vi "LSCI332ReadCalib.vi"(0 "VISA Rsrc":refnum<visa-resource-name>="GPIB0::12::INSTR" caption="Adresse du contrôlleur", 2 "No Courbe":u32=21 min=1 max=41 step=1, 11 "error in":errorcluster) -> (3 "Nom":string="CourbeTest", 4 "ValCalib":dbl[][](array[numeric]) caption="Valeurs de Calibration", 6 "No de série":string="Standard", 8 "Coefficient":u16(ring)=2 items=["Faites un choix", "négatif", "positif"], 10 "Format":u16(ring)=2 items=["Faites un choix", "mV/K", "V/K", "Ohm/K", "log Ohm/K"], 14 "TLim":dbl=475.0 caption="T° de Contrôle Max (K)", 15 "error out":errorcluster)   [LabVIEW 2012]
doc: "Ce Vi écrit l'entête et les points d'une courbe de calibration dans l'emplacement spécifié du contrôlleur de température"
panel:
  # "Température (K)"
  # "Sortie Capteur"
  # "+5"
  # "+10"
  # "+15"
  # "+20"
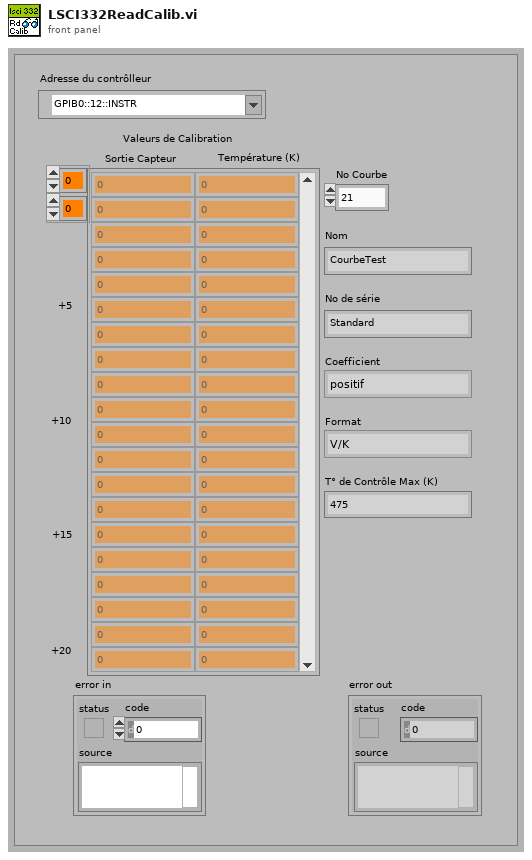
[diagram p1: front panel]
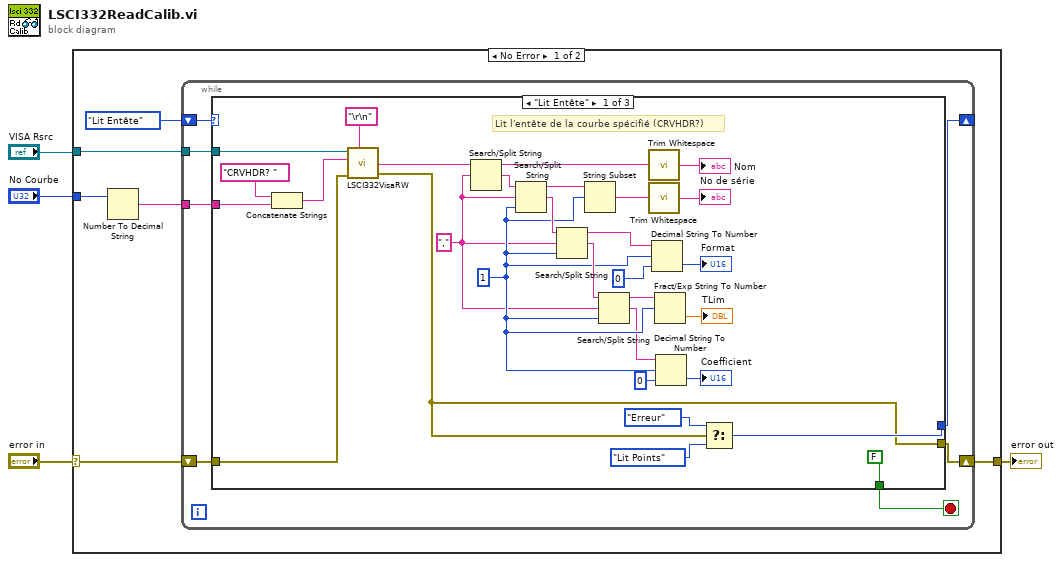
[diagram p0: block diagram]
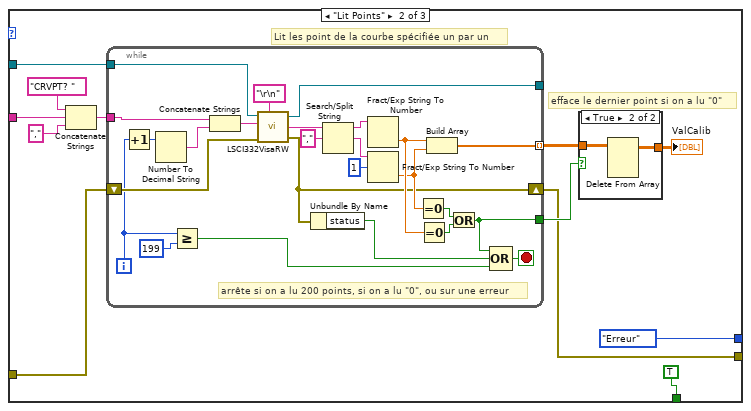
[diagram p2: hidden frame]
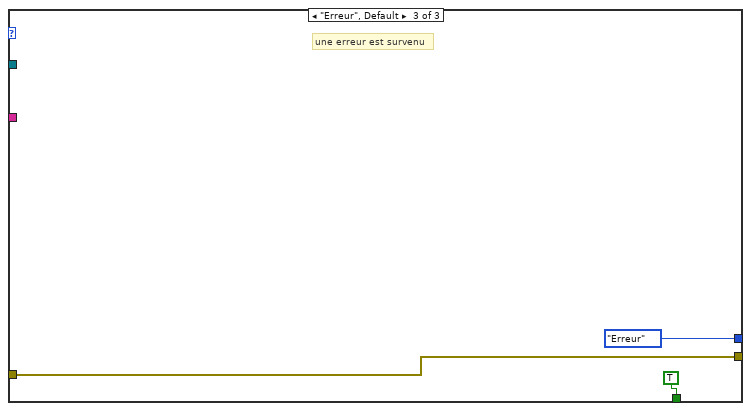
[diagram p4: hidden frame]
diagram:
  n1 = case shown="No Error" "error in" {
    selector: "error in" -> [w10 w91]
    tunnel: "VISA Rsrc" -> [w7 _]
    tunnel: "No Courbe" -> [w9 _]
    tunnel: [w6 w91] -> w1
    frame No Error {
      n2 = Number To Decimal String(number=w9) -> (decimal integer string=w8:string)  [unwired: 1 in]
      n3 = while {
        shift-right: [w11] -> w6
        shift-left: w10 -> [w17]
        tunnel: w8 -> [w15]
        tunnel: w7 -> [w14]
        shift-right: [w12] -> _
        shift-left: enum16{"Lit Entête", "Lit Points", "Erreur"}."Lit Entête" -> [w13]
        stop <- w16 stop-if-true
        n4 = case shown="\"Lit Entête\"" w13 {
          tunnel: w17 -> [w42 w54 w88]
          tunnel: [FALSE TRUE TRUE] -> w16
          tunnel: w15 -> [w45 w55 _]
          tunnel: w14 -> [w43 w56 _]
          tunnel: [w20 enum16{"Lit Entête", "Lit Points", "Erreur"}."Erreur" enum16{"Lit Entête", "Lit Points", "Erreur"}."Erreur"] -> w12
          tunnel: [w19 w50 w88] -> w11
          frame "Lit Entête" {
            w18 = ","
            w26 = 1
            # "Lit l'entête de la courbe spécifié (CRVHDR?)"
            n5 = Concatenate Strings("CRVHDR? ", w45) -> (w44:string)
            n6 = call <userlib>:"LSCI332VisaRW.vi"("error in (no error)"=w42, "EOS (Aucun)"="\r\n", "ChaineCom"=w44, "VISA Rsrc"=w43) -> ("error out"=w19:errorcluster, "ChaineRep"=w39:string)  [unwired: 3 in, 2 out]
            n7 = Search/Split String(string=w39, search string/char (-)=w18) -> (substring before match=w32:string, match + rest of string=w40:string)  [unwired: 1 in, 1 out]
            n8 = Search/Split String(string=w40, search string/char (-)=w18, offset (0)=w26) -> (substring before match=w38:string, match + rest of string=w41:string)  [unwired: 1 out]
            n9 = Search/Split String(string=w41, search string/char (-)=w18, offset (0)=w26) -> (substring before match=w37:string, match + rest of string=w34:string)  [unwired: 1 out]
            n10 = String Subset(string=w38, offset (0)=w26) -> (substring=w30:string)  [unwired: 1 in]
            n11 = Search/Split String(string=w34, search string/char (-)=w18, offset (0)=w26) -> (substring before match=w33:string, match + rest of string=w25:string)  [unwired: 1 out]
            n12 = call <vilib>:"Trim Whitespace.vi"("string"=w32) -> ("trimmed string"=→"Nom":string)  [unwired: 1 in]
            n13 = call <vilib>:"Trim Whitespace.vi"("string"=w30) -> ("trimmed string"=→"No de série":string)  [unwired: 1 in]
            n14 = Decimal String To Number(string=w37, offset=w26, default (0L)=u16 0 ("default (0 I32)")) -> (number=→"Format":u16)  [unwired: 1 out]
            n15 = Fract/Exp String To Number(string=w33, offset=w26) -> (number=→"TLim":dbl)  [unwired: 2 in, 1 out]
            n16 = Decimal String To Number(string=w25, offset=w26, default (0L)=u16 0 ("default (0 I32)")) -> (number=→"Coefficient":u16)  [unwired: 1 out]
            n17 = Select(t=enum16{"Lit Entête", "Lit Points", "Erreur"}."Erreur", s=w19, f=enum16{"Lit Entête", "Lit Points", "Erreur"}."Lit Points") -> (s? t:f=w20:enum16{"Lit Entête", "Lit Points", "Erreur"})
          }
          frame "Lit Points" {
            # "Lit les point de la courbe spécifiée un par un"
            # "efface le dernier point si on a lu \"0\""
            n18 = Concatenate Strings("CRVPT? ", w55, ",") -> (w58:string)
            n19 = while {
              tunnel: w58 -> [w87]
              tunnel: w56 -> [w85]
              shift-right: [w65] -> w50
              shift-left: w54 -> [w84]
              tunnel: [w71] -> w53 mode=indexing
              tunnel: [w77] -> _
              tunnel: [w66] -> w51
              i -> [w75]
              stop <- w72 stop-if-true
              # "arrête si on a lu 200 points, si on a lu \"0\", ou sur une erreur"
              n20 = Increment(x=w75) -> (x+1=w74:i32)
              n21 = Number To Decimal String(number=w74) -> (decimal integer string=w73:string)  [unwired: 1 in]
              n22 = Greater Or Equal?(x=w75, y=199) -> (x >= y?=w64:bool)
              n23 = Concatenate Strings(w87, w73) -> (w86:string)
              n24 = call <userlib>:"LSCI332VisaRW.vi"("error in (no error)"=w84, "EOS (Aucun)"="\r\n", "ChaineCom"=w86, "VISA Rsrc"=w85) -> ("error out"=w65:errorcluster, "ChaineRep"=w82:string, "VISA Rsrc Out"=w77:refnum<visa-resource-name>)  [unwired: 3 in, 1 out]
              n25 = Unbundle By Name(w65) -> ("status"=w63:bool)
              n26 = Search/Split String(string=w82, search string/char (-)=",") -> (substring before match=w80:string, match + rest of string=w79:string)  [unwired: 1 in, 1 out]
              n27 = Fract/Exp String To Number(string=w80) -> (number=w70:dbl)  [unwired: 3 in, 1 out]
              n28 = Fract/Exp String To Number(string=w79, offset=1) -> (number=w69:dbl)  [unwired: 2 in, 1 out]
              n29 = Equal To 0?(x=w69) -> (x = 0?=w67:bool)
              n30 = Equal To 0?(x=w70) -> (x = 0?=w68:bool)
              n31 = Build Array(w70, w69) -> (w71:dbl[])
              n32 = Or(x=w67, y=w68) -> (x .or. y?=w66:bool)
              n33 = Compound Arithmetic op=OR(w66, w63, w64) -> (w72:bool)
            }
            n34 = case shown="True" w51 {
              tunnel: w53 -> [w60 w62]
              tunnel: [w60 w61] -> w52
              frame False {
              }
              frame True {
                n35 = Delete From Array(array=w62) -> (array with subset deleted=w61:dbl[][])  [unwired: 3 in, 1 out]
              }
            }
            "ValCalib" <- w52
          }
          frame "Erreur", Default {
            # "une erreur est survenu"
          }
        }
      }
    }
    frame Error {
    }
  }
  "error out" <- w1
